vi "set Local Machine Ip Number.vi"(8 "error in":errorcluster, 11 "ipNumber":string) -> (0 "error out":errorcluster, 3 "ipNumber out":string)   [LabVIEW 2021, in "CycloneControlSDK.lvlib"]
doc: "extern \"C\" void _cdecl setLocalMachineIpNumber(char *ipNumber);"
uses:
  CycloneControlSDK.lvlib
  CycloneControlSDK_64.dll
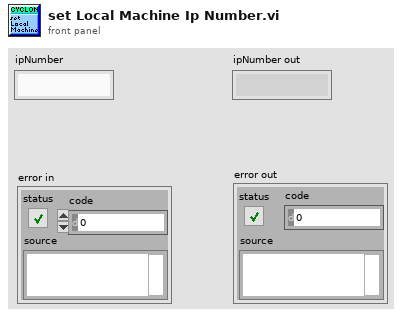
[diagram p1: front panel]
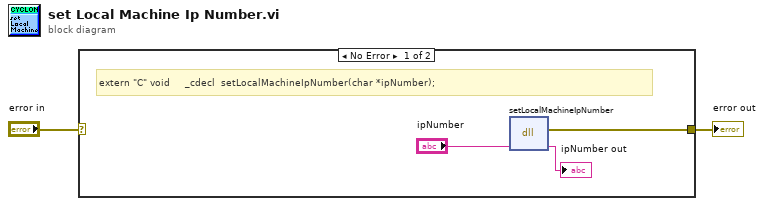
[diagram p0: block diagram]
diagram:
  n1 = case shown="No Error" "error in" {
    selector: "error in" -> [_ w6]
    tunnel: [w3 w6] -> w1
    frame No Error {
      # "extern \"C\" void     _cdecl  setLocalMachineIpNumber(char *ipNumber);"
      n2 = dll-call lib="C:/PEMicro/cyclone/cycloneControl/controlsdk/examples/labview2018/user.lib/CycloneControlSDK/CycloneControlSDK_64.dll" fn="setLocalMachineIpNumber"("ipNumber"="ipNumber") -> (error out=w3:errorcluster, "ipNumber"=→"ipNumber out":string)  [unwired: 4 in, 1 out]
    }
    frame Error {
    }
  }
  "error out" <- w1
